vi "Deploy Library and Shared Variables.vi"(8 "error in":errorcluster) -> (0 "error out":errorcluster)   [LabVIEW 2017, in "Shared Variables Library.lvlib"]
doc: "Deploys shared variables on the local network. \nShared variables must be depolyed, after creation, in order for them to be visible on the network."
uses:
  Shared Variables Library.lvlib
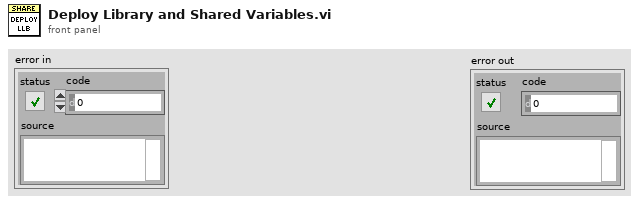
[diagram p1: front panel]
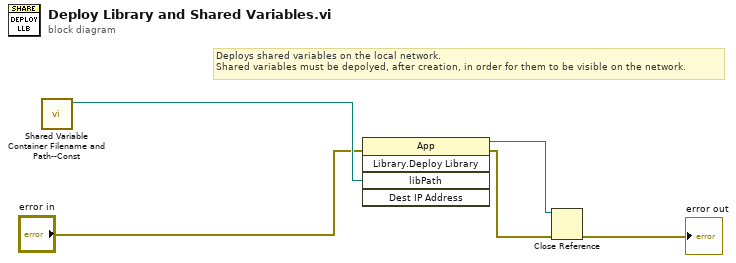
[diagram p0: block diagram]
diagram:
  # "Deploys shared variables on the local network. \nShared variables must be depolyed, after creation, in order for them to be visible on the network."
  n1 = call "Shared Variable Container Filename and Path--Const.vi"() -> ("Path to Shared Variable Containing Library"=w2:path)  [unwired: 11 in]
  n2 = invoke class="App" method="Library.Deploy Library"(error in="error in", "libPath"=w2) -> (reference out=w3:refnum<vi>, error out=w4:errorcluster)  [unwired: 3 in, 3 out]
  n3 = Close Reference(reference=w3, error in (no error)=w4) -> (error out=→"error out":errorcluster)
